vi "Autonomous Independent.vi"() -> ()   [LabVIEW 2014]
doc: "This VI is called when autonomous begins, and will automatically be terminated when autonomous ends. You can carry out timed or sensor driven robot movement independently without needing to return to the caller."
uses:
  Robot Global Data.vi
  <vilib>/Rock Robotics/WPI/RobotDrive/WPI_RobotDriveGetSetRefNum.vi
panel:
  out "error  out":errorcluster
  # "Be sure to right-click and choose Data Operations>>Make Current Value default if you want to save the array values with the VI"
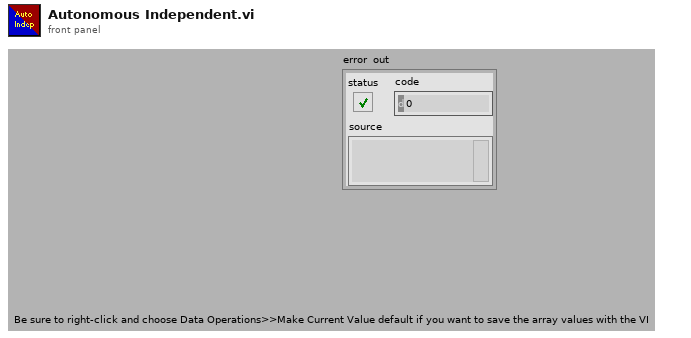
[diagram p1: front panel]
types:
  T1 = typedef "WPI_RobotDriveDevRef.ctl" = cluster{"DevStatus":errorcluster, "Motors[]":T2[], "Square Inputs":bool, "Max Output":dbl}
  T2 = typedef "WPI_MotorControlDeviceRef.ctl" = cluster{"DeviceStatus":errorcluster, "Type":enum16{"PWM", "CAN"}, "PWM":cluster{"Controller":T3, "PWM Channel":T4, "DeadBand":T5}, "CAN":cluster{"Device Number":u8, "Control Mode":T6, "Semaphore":T7, "Max Vout":dbl}, "Invert":bool, "TransformRef":T8, "InvTransformRef":T8}
  T3 = typedef "FPGA_TypedefDigitalModule.ctl" = enum16{"Controller 1"}
  T4 = typedef "FPGA_DIOPWMChannel.ctl" = enum8{"PWM 0", "PWM 1", "PWM 2", "PWM 3", "PWM 4", "PWM 5", "PWM 6", "PWM 7", "PWM 8", "PWM 9", "PWM MXP 0", "PWM MXP 1", "PWM MXP 2", "PWM MXP 3", "PWM MXP 4", "PWM MXP 5", "PWM MXP 6", "PWM MXP 7", "PWM MXP 8", "PWM MXP 9", "Invalid"}
  T5 = typedef "WPI_PWMDeadband.ctl" = cluster{"Name":string, "maxPositivePwm":i32, "minPositivePwm":i32, "centerPwm":i32, "maxNegativePwm":i32, "minNegativePwm":i32, "angularRange":u16}
  T6 = typedef "WPI_CANJaguar_ControlMode.ctl" = enum8{"Percent VBus", "Current", "Speed", "Position", "Voltage"}
  T7 = typedef "Semaphore RefNum" = refnum<k1>
  T8 = typedef "WPI_PWMTransform_ConPane.ctl" = refnum<vi>
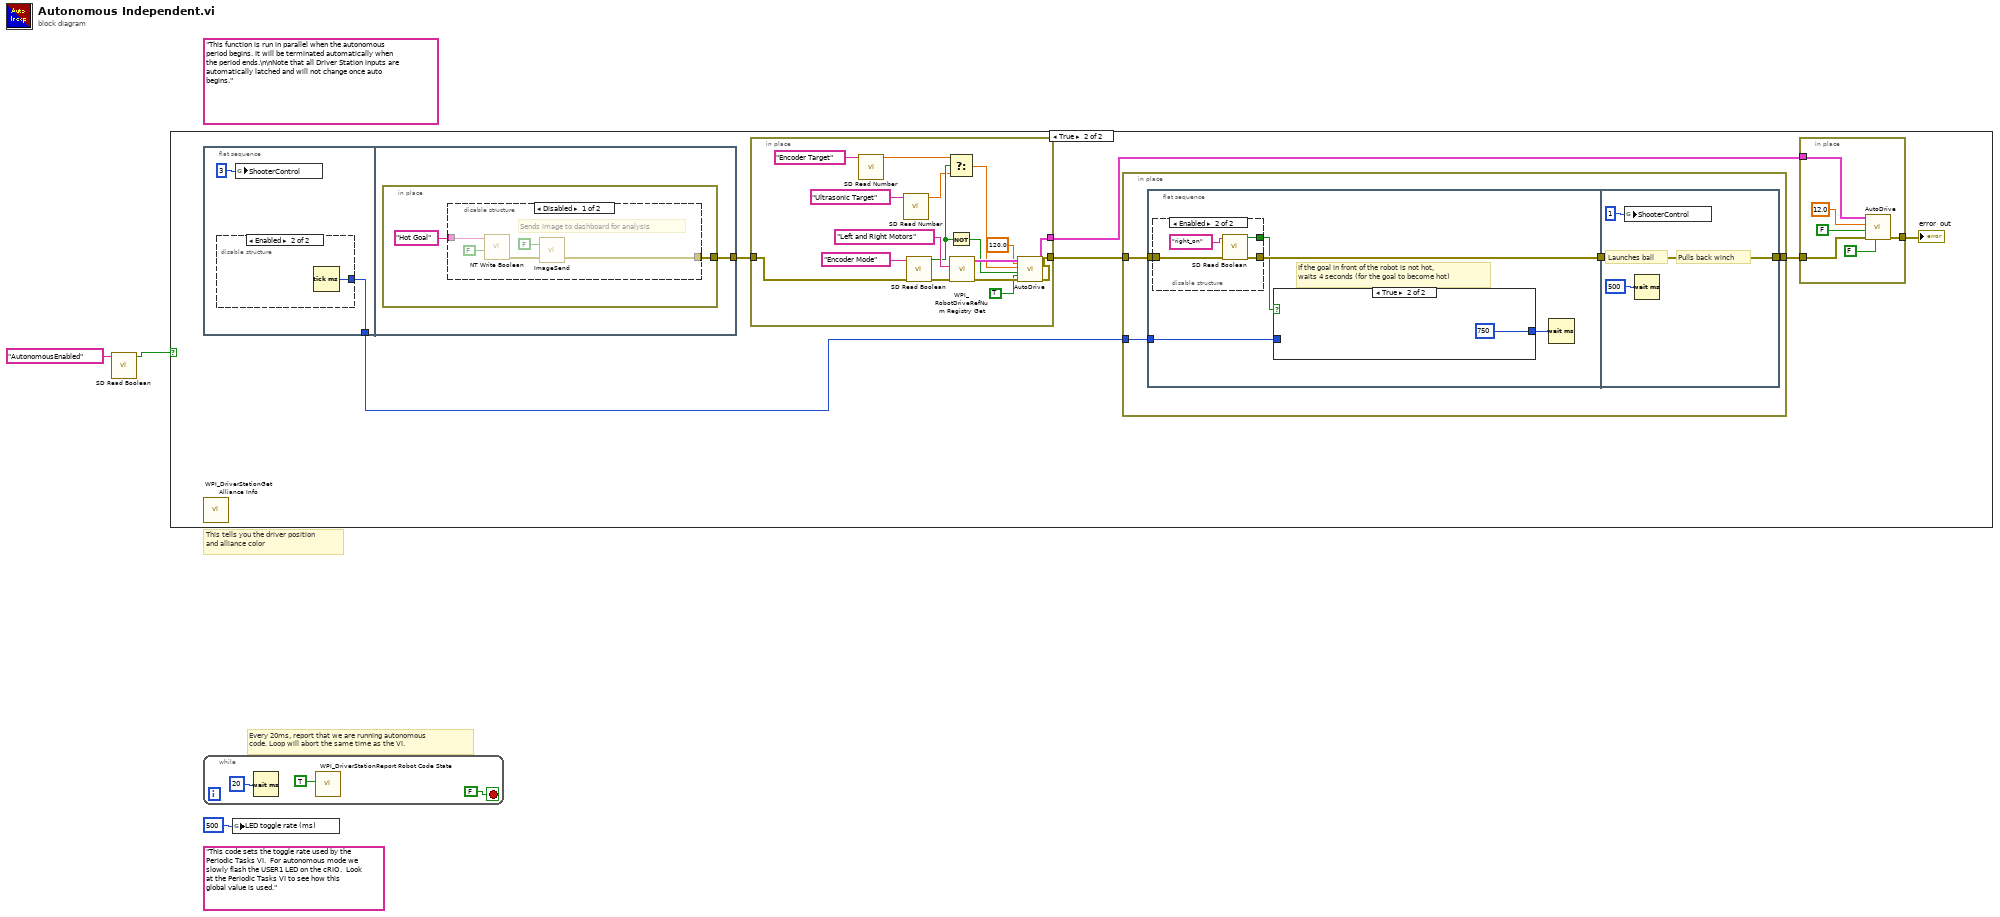
[diagram p0: block diagram]
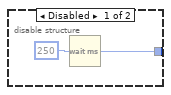
[diagram p3: hidden frame]
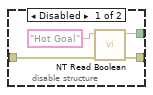
[diagram p5: hidden frame]
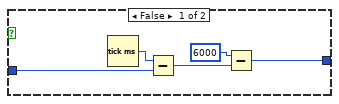
[diagram p6: hidden frame]
diagram:
  (unwired) "This function is run in parallel when the autonomous period begins. It will be terminated automatically when the period ends.\n\nNote that all Driver Station inputs are automatically latched and will not change once auto begins."
  (unwired) "This code sets the toggle rate used by the Periodic Tasks VI.  For autonomous mode we slowly flash the USER1 LED on the cRIO.  Look at the Periodic Tasks VI to see how this global value is used."
  # "Every 20ms, report that we are running autonomous\ncode. Loop will abort the same time as the VI."
  # "This tells you the driver position\nand alliance color"
  n1 = call <vilib>:"SD Read Boolean.vi"("Name"="AutonomousEnabled") -> ("Boolean"=w1:bool)  [unwired: 8 in, 2 out]
  n2 = case shown="True" w1 {
    frame False {
    }
    frame True {
      n3 = flat-sequence {
        tunnel: [w11] -> w6
        tunnel: [w15] -> w7
        frame #0 {
          n4 = disable-structure shown="Enabled" {
            disable-tunnel: [w12 w14] -> w11
            frame Disabled {
              n5 = Wait (ms)(milliseconds to wait=u32 250) -> (millisecond timer value=w12:u32)
            }
            frame Enabled {
              n6 = Tick Count (ms)() -> (millisecond timer value=w14:u32)
            }
          }
          n7 = global write "Robot Global Data.vi" "ShooterControl"(u32 3 ("ShooterControl")) -> ()
        }
        frame #1 {
          n8 = in-place {
            in-place-border: [w17] -> w15
            n9 = disable-structure shown="Disabled" {
              disable-tunnel: [w22 _] -> w17
              disable-tunnel: "Hot Goal" ("Name") -> [w19 _]
              frame Disabled {
                # "Sends image to dashboard for analysis"
                n10 = call <vilib>:"NT Write Boolean.vi"("Boolean"=FALSE, "Name"=w19) -> ("error out"=w20:errorcluster)  [unwired: 9 in]
                n11 = call "ImageSend.vi"("error in (no error)"=w20, "mode (T=AutoAim, F=HotGoal)"=FALSE) -> ("error out"=w22:errorcluster)  [unwired: 1 in]
              }
              frame Enabled {
              }
            }
          }
        }
      }
      n12 = call <vilib>:"WPI_DriverStationGet Alliance Info.vi"() -> ()  [unwired: 12 out]
      n13 = in-place {
        in-place-border: [w68] -> w9
        in-place-border: [w67] -> w5
        in-place-border: w7 -> [w63]
        n14 = call <vilib>:"SD Read Number.vi"("Name"="Encoder Target") -> ("Numeric"=w56:dbl)  [unwired: 8 in, 2 out]
        n15 = call <vilib>:"SD Read Number.vi"("Name"="Ultrasonic Target") -> ("Numeric"=w57:dbl)  [unwired: 8 in, 2 out]
        n16 = call <vilib>:"SD Read Boolean.vi"("error in"=w63, "Name"="Encoder Mode") -> ("error out"=w62:errorcluster, "Boolean"=w60:bool)  [unwired: 7 in, 1 out]
        n17 = Select(t=w56, s=w60, f=w57) -> (s? t:f=w59:dbl)
        n18 = Not(x=w60) -> (.not. x?=w55:bool)
        n19 = call <vilib>:"WPI_RobotDriveRefNum Registry Get.vi"("error in (no error)"=w62, "refnum name"="Left and Right Motors") -> ("error out"=w69:errorcluster, "RobotDriveDevRef"=w70:T1)  [unwired: 8 in]
        n20 = call "AutoDrive.vi"("Reset"=TRUE ("Forwards"), "Distance before ultrasonic PID"=120.0, "error in (no error)"=w69, "mode(T:ultrasonic,F:encoders)"=w55, "target"=w59, "RobotDriveDevRef"=w70) -> ("error out"=w67:errorcluster, "RobotDriveDevRef"=w68:T1)  [unwired: 4 in]
      }
      n21 = in-place {
        in-place-border: w5 -> [w25]
        in-place-border: [w26] -> w8
        in-place-border: w6 -> [w23]
        n22 = flat-sequence {
          tunnel: w25 -> [w29]
          tunnel: [w28] -> w24
          tunnel: w23 -> [w31]
          tunnel: [w48] -> w26
          tunnel: w24 -> [w48]
          frame #0 {
            # "If the goal in front of the robot is not hot,\nwaits 4 seconds (for the goal to become hot)"
            n23 = disable-structure shown="Enabled" {
              disable-tunnel: w29 -> [w35 w37]
              disable-tunnel: [w34 w39] -> w28
              disable-tunnel: [w32 w36] -> w27
              frame Disabled {
                n24 = call <vilib>:"NT Read Boolean.vi"("error in"=w35, "Name"="Hot Goal") -> ("error out"=w34:errorcluster, "Boolean"=w32:bool)  [unwired: 8 in]
              }
              frame Enabled {
                n25 = call <vilib>:"SD Read Boolean.vi"("error in"=w37, "Name"="right_on") -> ("error out"=w39:errorcluster, "Boolean"=w36:bool)  [unwired: 7 in, 1 out]
              }
            }
            n26 = case shown="True" w27 {
              tunnel: w31 -> [w41 _]
              tunnel: [w40 u32 750 ("wait")] -> w30
              frame False {
                n27 = Tick Count (ms)() -> (millisecond timer value=w42:u32)
                n28 = Subtract(x=w42, y=w41) -> (x-y=w43:u32)
                n29 = Subtract(x=u32 6000, y=w43) -> (x-y=w40:u32)
              }
              frame True {
              }
            }
            n30 = Wait (ms)(milliseconds to wait=w30) -> ()  [unwired: 1 out]
          }
          frame #1 {
            # "Pulls back winch"
            # "Launches ball"
            n31 = global write "Robot Global Data.vi" "ShooterControl"(u32 1 ("ShooterControl")) -> ()
            n32 = Wait (ms)(milliseconds to wait=u32 500) -> ()  [unwired: 1 out]
          }
        }
      }
      n33 = in-place {
        in-place-border: w9 -> [w54]
        in-place-border: w8 -> [w53]
        in-place-border: [w52] -> w4
        n34 = call "AutoDrive.vi"("Reset"=FALSE ("Forwards"), "error in (no error)"=w53, "mode(T:ultrasonic,F:encoders)"=FALSE, "target"=12.0, "RobotDriveDevRef"=w54) -> ("error out"=w52:errorcluster)  [unwired: 5 in, 1 out]
      }
      "error  out" <- w4
    }
  }
  n35 = while {
    stop <- FALSE stop-if-true
    n36 = Wait (ms)(milliseconds to wait=u32 20) -> ()  [unwired: 1 out]
    n37 = call <vilib>:"WPI_DriverStationReport Robot Code State.vi"("Autonomous"=TRUE) -> ()  [unwired: 10 in, 1 out]
  }
  n38 = global write "Robot Global Data.vi" "LED toggle rate (ms)"(u32 500 ("LED ms toggle rate")) -> ()
